vi "openeod_working.vi"(8 "error in (no error)":errorcluster, 10 "size (in bytes)":i64, 11 "Byte Stream File in":refnum<file>) -> (0 "error out":errorcluster, 1 "EODDataOut":T1(array[cluster]), 2 "Iteration Number":i32, 3 "Byte Stream File out":refnum<file>)   [LabVIEW 2014]
panel:
  out "Wave Offset":i32[](array[numeric])
  # "EOD File Reader VI"
  # "Inputs"
  # "Outputs"
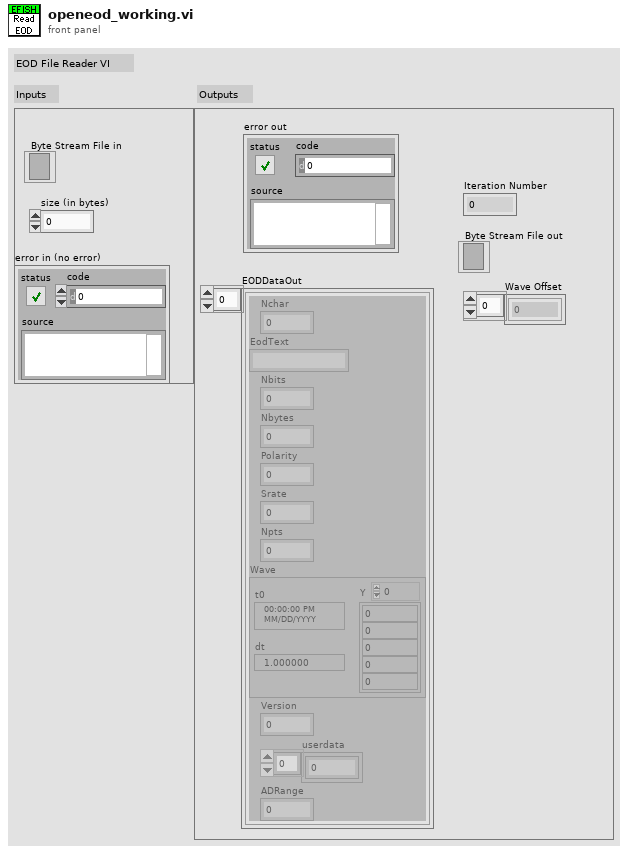
[diagram p1: front panel]
types:
  T1 = cluster{"Nchar":i32, "EodText":string, "Nbits":i32, "Nbytes":i32, "Polarity":i32, "Srate":i32, "Npts":i32, "Wave":waveform(dbl), "Version":i32, "userdata":dbl[], "ADRange":dbl}[]
  T2 = cluster{"Nchar":i32, "EodText":string, "Nbits":i32, "Nbytes":i32, "Polarity":i32, "Srate":i32, "Npts":i32, "Wave":waveform(dbl), "Version":i32, "userdata":dbl[], "ADRange":dbl}
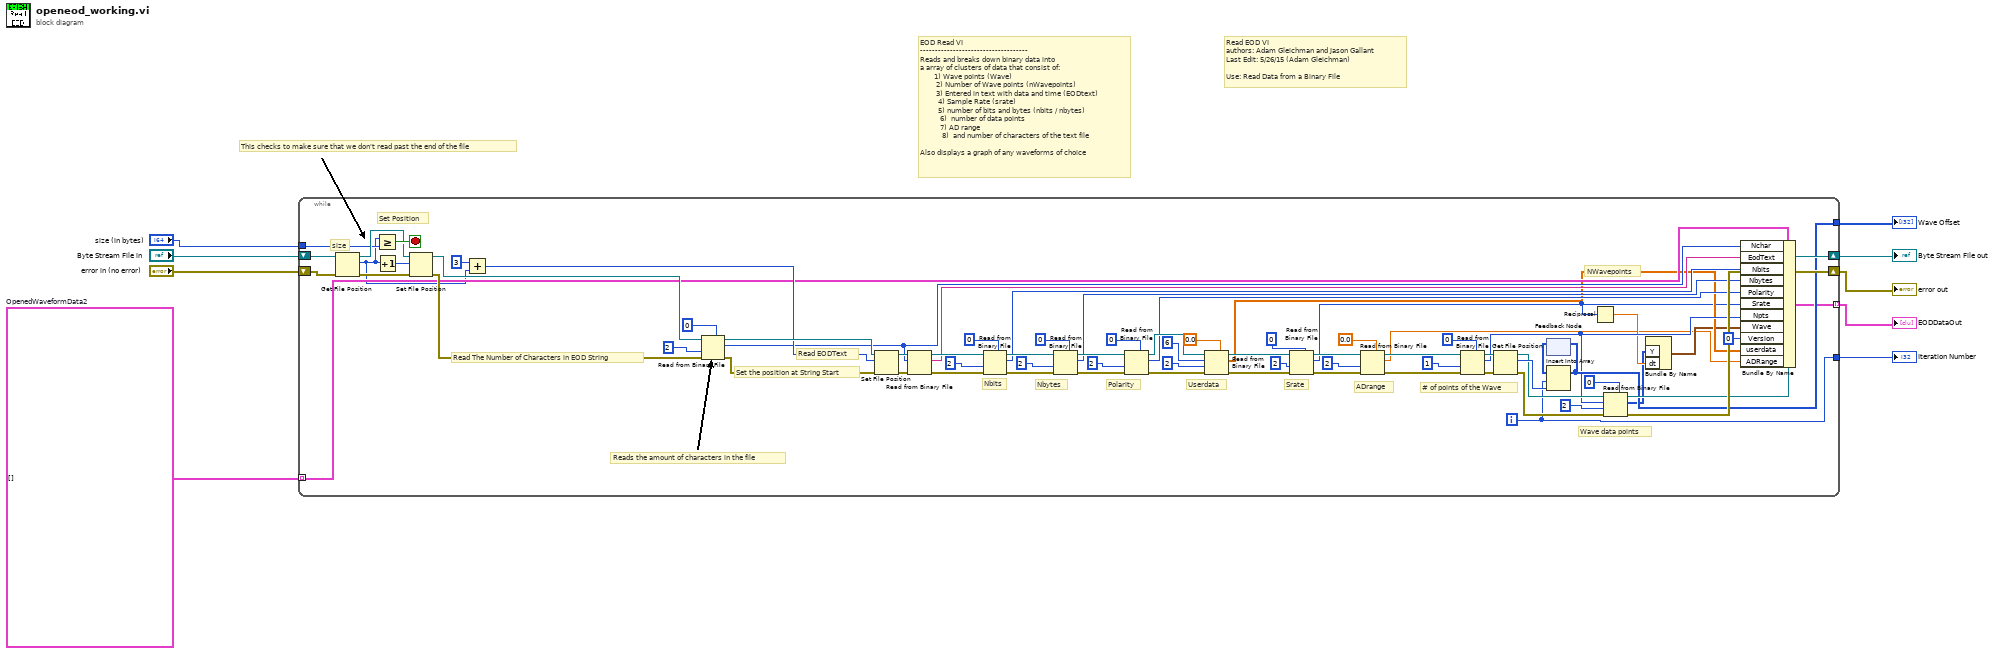
[diagram p0: block diagram]
diagram:
  w2 = T1 []  # OpenedWaveformData2
  # "Read EOD VI\nauthors: Adam Gleichman and Jason Gallant\nLast Edit: 5/26/15 (Adam Gleichman)\n\nUse: Read Data from a Binary File"
  # "This checks to make sure that we don't read past the end of the file"
  # "EOD Read VI\n------------------------------------\nReads and breaks down binary data into\na array of clusters of data that consist of:\n       1) Wave points (Wave)\n        2) Number of Wave points (nWavepoints)\n        3) Entered in text with data and time (EODtext)\n         4) Sample Rate (srate) \n         5) number of bits and bytes (nbits / nbytes)\n          6)  number of data points\n          7) AD range\n           8)  and number of characters of the text file\n\nAlso displays a graph of any waveforms of choice"
  n1 = while {
    shift-right: [w34] -> w7
    shift-left: "Byte Stream File in" -> [w43]
    shift-right: [w39] -> w8
    shift-left: "error in (no error)" -> [w40]
    tunnel: "size (in bytes)" -> [w36]
    tunnel: [w27] -> w6
    tunnel: [w26] -> w3
    tunnel: w2 -> [w25] mode=indexing
    tunnel: [w12] -> w1 mode=indexing
    i -> [w27]
    stop <- w44 stop-if-true
    # "ADrange"
    # "Nbits"
    # "Reads the amount of characters in the file"
    # "size"
    # "# of points of the Wave"
    # "Wave data points"
    # "NWavepoints"
    # "Srate"
    # "Userdata"
    # "Polarity"
    # "Nbytes"
    # "Read EODText"
    # "Set the position at String Start"
    # "Read The Number of Characters in EOD String"
    # "Set Position"
    n2 = Get File Position(4:w40, 7:w43) -> (0:w41:errorcluster, 2:w10:i64, 3:w42:refnum<file>)
    n3 = Greater Or Equal?(x=w10, y=w36) -> (x >= y?=w44:bool)
    n4 = Increment(x=w10) -> (x+1=w35:i64)
    n5 = Set File Position(offset (in bytes) (0)=w35, refnum=w42, error in=w41) -> (refnum out=w82:refnum<file>, error out=w54:errorcluster)  [unwired: 1 in]
    n6 = Add(x=3, y=w10) -> (x+y=w38:i64)
    n7 = Read from Binary File(5:u8 0, 8:w54, 9:2, 11:w82) -> (0:w53:errorcluster, 2:w22:u8, 3:w81:refnum<file>)  [unwired: 2 in, 1 out]
    n8 = Set File Position(offset (in bytes) (0)=w38, refnum=w81, error in=w53) -> (refnum out=w80:refnum<file>, error out=w52:errorcluster)  [unwired: 1 in]
    n9 = Read from Binary File(8:w52, 10:w22, 11:w80) -> (0:w51:errorcluster, 2:w23:string, 3:w79:refnum<file>)  [unwired: 3 in, 1 out]
    n10 = Read from Binary File(5:i8 0, 8:w51, 9:2, 11:w79) -> (0:w50:errorcluster, 2:w21:i8, 3:w56:refnum<file>)  [unwired: 2 in, 1 out]
    n11 = Read from Binary File(5:i8 0, 8:w50, 9:2, 11:w56) -> (0:w49:errorcluster, 2:w20:i8, 3:w57:refnum<file>)  [unwired: 2 in, 1 out]
    n12 = Read from Binary File(5:i8 0, 8:w49, 9:2, 11:w57) -> (0:w48:errorcluster, 2:w19:i8, 3:w55:refnum<file>)  [unwired: 2 in, 1 out]
    n13 = Read from Binary File(5:sgl 0.0, 8:w48, 9:2, 10:6, 11:w55) -> (0:w47:errorcluster, 2:w18:sgl[], 3:w76:refnum<file>)  [unwired: 1 in, 1 out]
    n14 = Read from Binary File(5:u32 0, 8:w47, 9:2, 11:w76) -> (0:w46:errorcluster, 2:w17:u32, 3:w68:refnum<file>)  [unwired: 2 in, 1 out]
    n15 = Read from Binary File(5:sgl 0.0, 8:w46, 9:2, 11:w68) -> (0:w45:errorcluster, 2:w13:sgl, 3:w63:refnum<file>)  [unwired: 2 in, 1 out]
    n16 = Read from Binary File(5:u32 0, 8:w45, 9:1, 11:w63) -> (0:w29:errorcluster, 2:w24:u32, 3:w31:refnum<file>)  [unwired: 2 in, 1 out]
    n17 = Get File Position(4:w29, 7:w31) -> (0:w28:errorcluster, 2:w33:i64, 3:w30:refnum<file>)
    n18 = feedback #1() -> (w32:i64[])  [unwired: 1 in]
    n19 = Insert Into Array(array=w32, index=w27, new element=w33) -> (w26:i64[])
    n20 = feedback-in #1(w26) -> ()
    n21 = Reciprocal(x=w17) -> (1/x=w16:dbl)
    n22 = Read from Binary File(5:i16 0, 8:w28, 9:2, 10:w24, 11:w30) -> (0:w39:errorcluster, 2:w15:i16[], 3:w34:refnum<file>)  [unwired: 1 in, 1 out]
    n23 = Bundle By Name("Y"=w15, "dt"=w16) -> (w14:waveform(i16))  [unwired: 1 in]
    n24 = Bundle By Name(cluster=w25, "Nchar"=w22, "EodText"=w23, "Nbits"=w21, "Nbytes"=w20, "Polarity"=w19, "Srate"=w17, "Npts"=w24, "Wave"=w14, "Version"=0, "userdata"=w18, "ADRange"=w13) -> (w12:T2)
  }
  "error out" <- w8
  "Byte Stream File out" <- w7
  "Iteration Number" <- w6
  "Wave Offset" <- w3
  "EODDataOut" <- w1
